vi "扭矩标定.vi"(11 "输入扭矩":dbl) -> (3 "输出百分比":dbl)   [LabVIEW 2016]
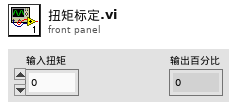
[diagram p1: front panel]
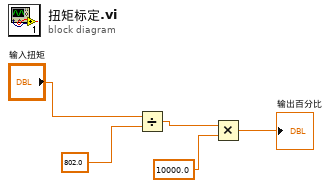
[diagram p0: block diagram]
diagram:
  n1 = Divide(x="输入扭矩", y=802.0) -> (x/y=w3:dbl)
  n2 = Multiply(x=w3, y=10000.0) -> (x*y=→"输出百分比":dbl)
